vi "ASCII CMD-Response Instrument.vi"() -> ()   [LabVIEW 2019]
uses:
  <vilib>/numeric/Random Number (Range) DBL.vi
  <vilib>/Instr/_visa.llb/VISA Configure Serial Port (Instr).vi
panel:
  out "read buffer":string
  out "error out":errorcluster
  in  "stop":bool
  in  "VISA resource name":refnum<visa-resource-name>
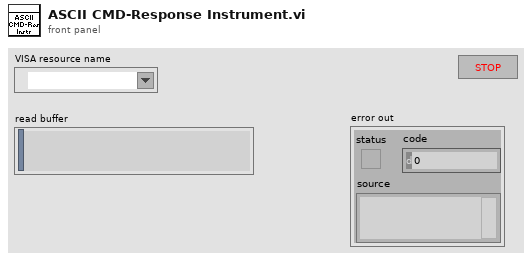
[diagram p1: front panel]
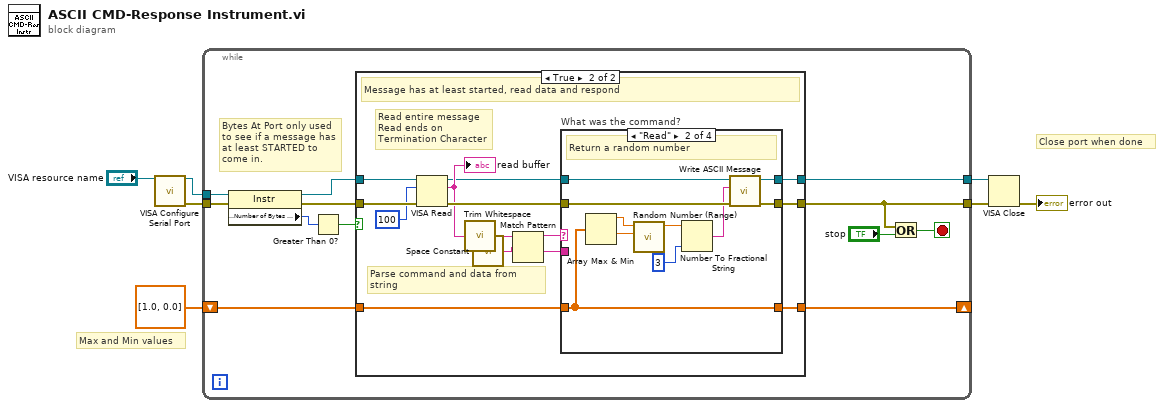
[diagram p0: block diagram]
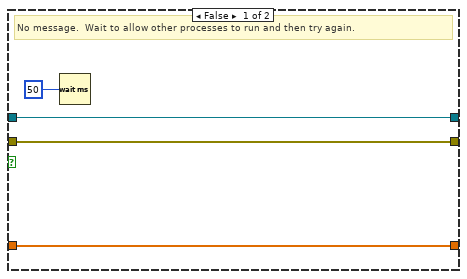
[diagram p2: hidden frame]
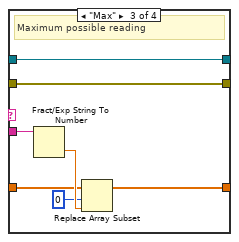
[diagram p4: hidden frame]
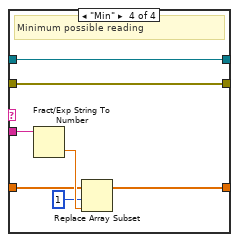
[diagram p5: hidden frame]
diagram:
  # "Max and Min values"
  # "Close port when done"
  n1 = call-poly "VISA Configure Serial Port"("VISA resource name"="VISA resource name") -> ("VISA resource name out"=w2:refnum<visa-resource-name>, "error out"=w5:errorcluster)  [unwired: 13 in]
  n2 = while {
    tunnel: w5 -> [w19]
    tunnel: w2 -> [w16]
    tunnel: [w12] -> w3
    tunnel: [w17] -> w7
    shift-right: [w8] -> _
    shift-left: dbl[] [1.0, 0.0] -> [w9]
    stop <- w11 stop-if-true
    # "Bytes At Port only used\nto see if a message has\nat least STARTED to\ncome in."
    n3 = property class="Instr"(reference=w16, error in=w19) -> (reference out=w13:refnum<visa-resource-name>, error out=w18:errorcluster, "Serial Settings:Number of Bytes at Serial Port"=w15:u32)
    n4 = Greater Than 0?(x=w15) -> (x > 0?=w14:bool)
    n5 = case shown="True" w14 {
      tunnel: w18 -> [w23 w37]
      tunnel: w13 -> [w22 w34]
      tunnel: [w22 w29] -> w12
      tunnel: [w23 w35] -> w17
      tunnel: w9 -> [w20 w30]
      tunnel: [w20 w28] -> w8
      frame False {
        # "No message.  Wait to allow other processes to run and then try again."
        n6 = Wait (ms)(milliseconds to wait=u32 50) -> ()  [unwired: 1 out]
      }
      frame True {
        # "Parse command and data from string"
        # "Read entire message\nRead ends on\nTermination Character"
        # "Message has at least started, read data and respond"
        n7 = VISA Read(VISA resource name=w34, byte count=u32 100, error in (no error)=w37) -> (VISA resource name out=w31:refnum<visa-resource-name>, read buffer=w33:string, error out=w36:errorcluster)  [unwired: 1 out]
        "read buffer" <- w33
        n8 = call <vilib>:"Trim Whitespace.vi"("string"=w33) -> ("trimmed string"=w27:string)  [unwired: 1 in]
        n9 = call <vilib>:"Space Constant.vi"() -> ("String"=w24:string)
        n10 = Match Pattern(string=w27, regular expression=w24) -> (before substring=w26:string, after substring=w25:string)  [unwired: 1 in, 2 out]
        n11 = case "What was the command?" shown="\"Read\"" w26 {
          tunnel: w31 -> [w39 w47 w55 w62]
          tunnel: w36 -> [w40 w50 w57 w64]
          tunnel: w30 -> [w38 w41 w53 w60]
          tunnel: [w39 w44 w55 w62] -> w29
          tunnel: [w40 w49 w57 w64] -> w35
          tunnel: [w38 w41 w54 w61] -> w28
          tunnel: w25 -> [_ _ w52 w59]
          frame Default {
            # "Unknown command"
          }
          frame "Read" {
            # "Return a random number"
            n12 = Array Max & Min(array=w41) -> (max value=w43:dbl, min value=w42:dbl)  [unwired: 2 out]
            n13 = call-poly <vilib>:"Random Number (Range).vi"("lower bound (0)"=w42, "upper bound (100)"=w43) -> ("number"=w46:dbl)  [unwired: 9 in]
            n14 = Number To Fractional String(number=w46, precision (6)=i16 3) -> (F-format string=w45:string)  [unwired: 2 in]
            n15 = call "Write ASCII Message.vi"("error in"=w50, "Message"=w45, "VISA resource in"=w47) -> ("error out"=w49:errorcluster, "VISA resource out"=w44:refnum<visa-resource-name>)  [unwired: 7 in]
          }
          frame "Max" {
            # "Maximum possible reading"
            n16 = Fract/Exp String To Number(string=w52) -> (number=w56:dbl)  [unwired: 3 in, 1 out]
            n17 = Replace Array Subset(array=w53, new element=w56, index=0) -> (w54:dbl[])
          }
          frame "Min" {
            # "Minimum possible reading"
            n18 = Fract/Exp String To Number(string=w59) -> (number=w63:dbl)  [unwired: 3 in, 1 out]
            n19 = Replace Array Subset(array=w60, new element=w63, index=1) -> (w61:dbl[])
          }
        }
      }
    }
    n20 = Or(x=w17, y="stop") -> (x .or. y?=w11:bool)
  }
  n21 = VISA Close(VISA resource name=w3, error in (no error)=w7) -> (error out=→"error out":errorcluster)
